vi "BarcodeScan.vi"(6 "Model ME79? (T-ME79)":bool=TRUE, 11 "Barcode In":string) -> (1 "NG":bool, 3 "OK":bool)   [LabVIEW 2018]
panel:
  in  "Clear":bool
  in  "Cancel":bool
  in  "OK":bool
  in  "Barcode":string
  # "PLEASE SCAN BARCODE"
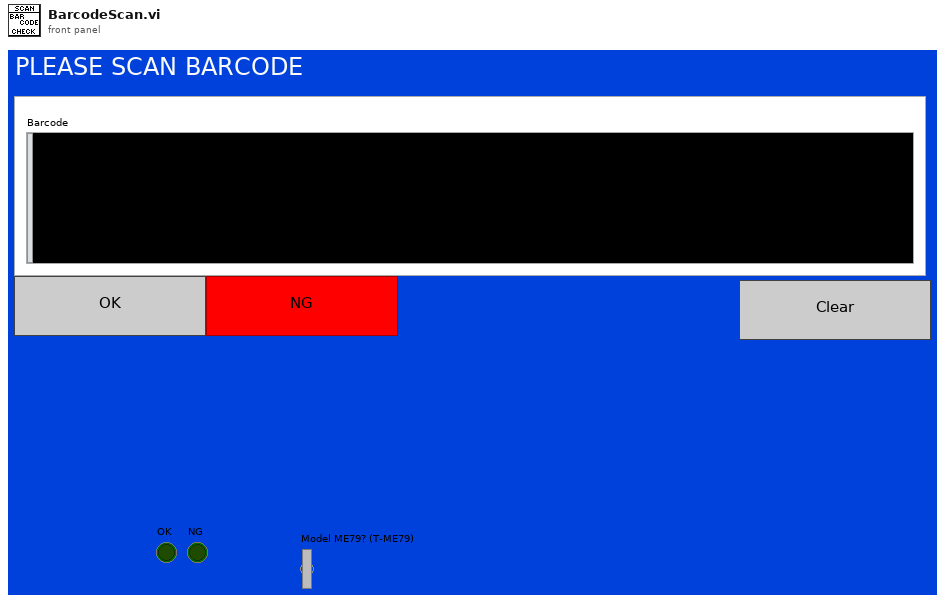
[diagram p1: front panel]
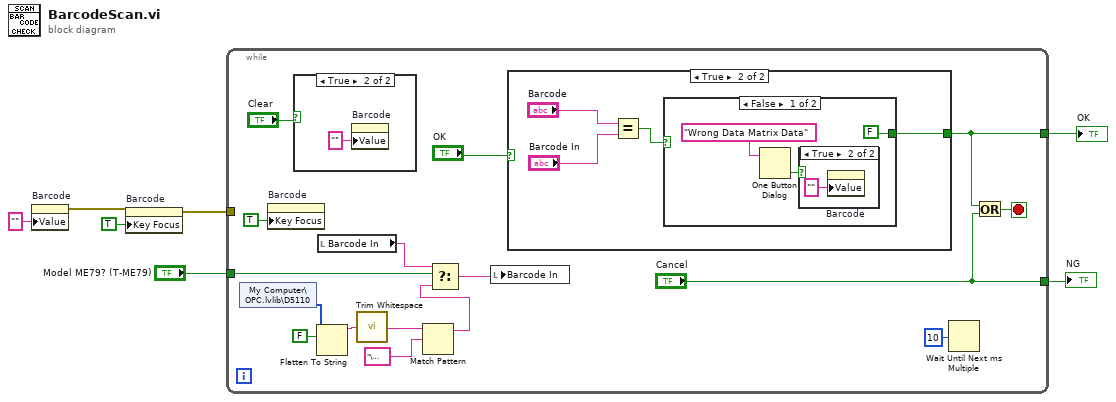
[diagram p0: block diagram]
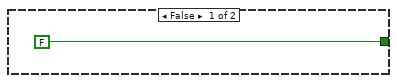
[diagram p2: hidden frame]
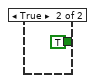
[diagram p4: hidden frame]
diagram:
  n1 = property on="Barcode" class="Str"("Value"="" ("Barcode")) -> (error out=w6:errorcluster)  [unwired: 2 in, 1 out]
  n2 = property on="Barcode" class="Str"(error in=w6, "Key Focus"=TRUE) -> (error out=w4:errorcluster)  [unwired: 1 in, 1 out]
  n3 = while {
    tunnel: w4 -> [_]
    tunnel: [w19] -> w3
    tunnel: ["Cancel"] -> w2
    tunnel: "Model ME79? (T-ME79)" -> [w16]
    stop <- w23 stop-if-true
    n4 = shared-variable "My Computer\\OPC.lvlib\\D5110"() -> (w13:u16[])  [unwired: 1 in, 1 out]
    n5 = property on="Barcode" class="Str"("Key Focus"=TRUE) -> ()  [unwired: 2 in, 2 out]
    n6 = case shown="True" "Clear" {
      frame False {
      }
      frame True {
        n7 = property on="Barcode" class="Str"("Value"="" ("Barcode")) -> ()  [unwired: 2 in, 2 out]
      }
    }
    n8 = Flatten To String(anything=w13, prepend array or string size? (T)=FALSE) -> (data string=w14:string)  [unwired: 2 in, 2 out]
    n9 = local read "Barcode In"() -> (w11:string)
    n10 = call <vilib>:"Trim Whitespace.vi"("string"=w14) -> ("trimmed string"=w10:string)  [unwired: 1 in]
    n11 = Match Pattern(string=w10, regular expression="\u0000") -> (before substring=w8:string)  [unwired: 1 in, 3 out]
    n12 = Select(t=w11, s=w16, f=w8) -> (s? t:f=w12:string)
    n13 = local write "Barcode In"(w12) -> ()
    n14 = case shown="True" "OK" {
      tunnel: [FALSE w26] -> w19
      frame False {
      }
      frame True {
        n15 = Equal?(x="Barcode", y="Barcode In") -> (x = y?=w27:bool)
        n16 = case shown="False" w27 {
          tunnel: [FALSE TRUE] -> w26
          frame False {
            n17 = One Button Dialog(message="Wrong Data Matrix Data") -> (true=w29:bool)  [unwired: 1 in]
            n18 = case shown="True" w29 {
              frame False {
              }
              frame True {
                n19 = property on="Barcode" class="Str"("Value"="" ("Barcode")) -> ()  [unwired: 2 in, 2 out]
              }
            }
          }
          frame True {
          }
        }
      }
    }
    n20 = Wait Until Next ms Multiple(millisecond multiple=u32 10 ("milliseconds to wait")) -> ()  [unwired: 1 out]
    n21 = Or(x=w19, y="Cancel") -> (x .or. y?=w23:bool)
  }
  "OK" <- w3
  "NG" <- w2
